vi "Write Resistor.vi"(8 "error in (no error)":errorcluster, 10 "Resistor Engine Refs in":T1 {"RT IDs"."Slot #" max=15; "RT IDs"."Chip Address (A2 A1 A0)" max=7; "RT Block Data Refs"."Data Reference" format="%.0x"}, 11 "DMA FIFO Ref in":refnum<k20>) -> (0 "error out":errorcluster, 2 "Resistor Engine Refs out":T1 {"RT IDs"."Slot #" max=15; "RT IDs"."Chip Address (A2 A1 A0)" max=7; "RT Block Data Refs"."Data Reference" format="%.0x"}, 3 "DMA FIFO Ref out":refnum<k20>)   [LabVIEW 2014, in "SLSC configuration Engine.lvlib"]
uses:
  SLSC configuration Engine.lvlib
  Type Defs/RT Engine Refs.ctl
  Shared/Type Defs/RT IDs.ctl
  Shared/SPI Utility/Slot #.ctl
  Shared/MCP23S17/Chip Address.ctl
  <vilib>/NI Veristand/Custom Device API/Block Data Reference.ctl
  <vilib>/NI Veristand/Custom Device API/Data Reference.ctl
  <vilib>/NI Veristand/Custom Device API/Global Data Refs.vi
  <vilib>/Utility/error.llb/Error Cluster From Error Code.vi
  <vilib>/rvi/errors/niLvFpgaAdjustHostInterfaceError.vi
  <vilib>/rvi/interface/nirviMethod/nirviMethod.xnode
  <vilib>/NI Veristand/Custom Device API/Custom Device API.lvlib
  <vilib>/FPGAPlugInAG/Dynamic/niLvFpga_WriteFifo_Dynamic.vi
  <vilib>/rvi/errors/niLvFpgaMergeErrorWithErrorCode.vi
  Shared/SLSC configuration Shared.lvlib
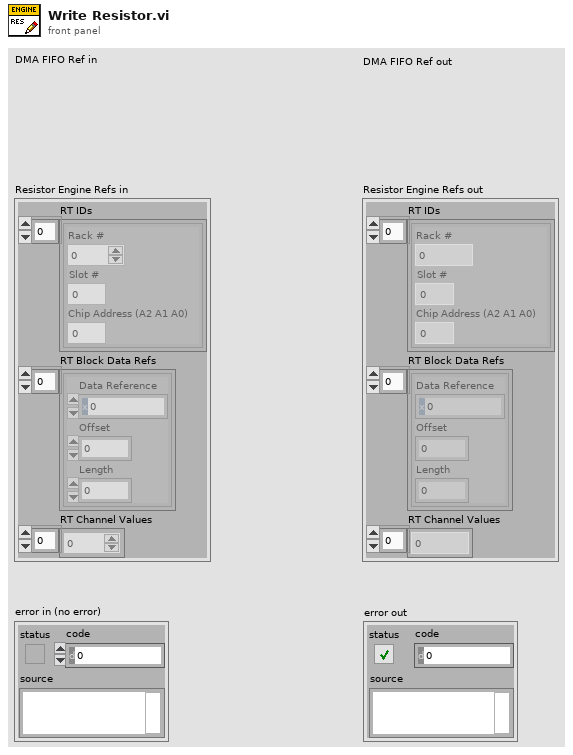
[diagram p1: front panel]
types:
  T1 = typedef "SLSC configuration Engine.lvlib/RT Engine Refs.ctl" = cluster{"RT IDs":T2[], "RT Block Data Refs":T5[], "RT Channel Values":dbl[]}
  T2 = typedef "SLSC configuration Shared.lvlib/RT IDs.ctl" = cluster{"Rack #":u8, "Slot #":T3, "Chip Address (A2 A1 A0)":T4}
  T3 = typedef "SLSC configuration Shared.lvlib/Slot #.ctl" = u8
  T4 = typedef "SLSC configuration Shared.lvlib/Chip Address.ctl" = u8
  T5 = typedef "Custom Device API.lvlib/Block Data Reference.ctl" = cluster{"Data Reference":T6, "Offset":i32, "Length":i32}
  T6 = typedef "Custom Device API.lvlib/Data Reference.ctl" = i32
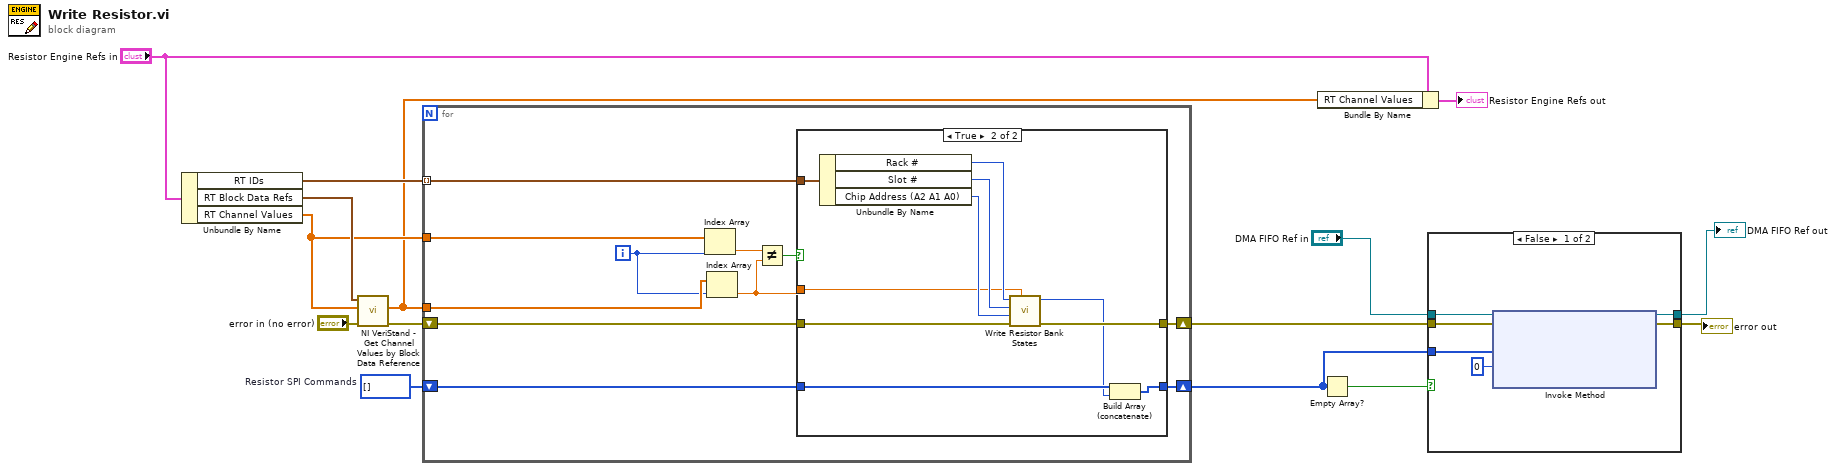
[diagram p0: block diagram]
diagram:
  w7 = u64[] []  # Resistor SPI Commands
  n1 = Unbundle By Name("Resistor Engine Refs in") -> ("RT IDs"=w12:T2[], "RT Block Data Refs"=w15:T5[], "RT Channel Values"=w10:dbl[])
  n2 = call <vilib>:"NI VeriStand - Get Channel Values by Block Data Reference.vi"("error in (no error)"="error in (no error)", "Values Array in"=w10, "Block Data Ref"=w15) -> ("error out"=w13:errorcluster, "Values Array out"=w9:dbl[])  [unwired: 6 in, 1 out]
  n3 = for {
    shift-right: [w20] -> w6
    shift-left: w13 -> [w22]
    tunnel: w12 -> [w23] mode=indexing
    tunnel: w9 -> [w25]
    tunnel: w10 -> [w26]
    shift-right: [w17] -> w3
    shift-left: w7 -> [w18]
    i -> [w16]
    n4 = Index Array(array=w26, index=w16) -> (element=w24:dbl)
    n5 = Index Array(array=w25, index=w16) -> (element=w21:dbl)
    n6 = Not Equal?(x=w24, y=w21) -> (x != y?=w19:bool)
    n7 = case shown="True" w19 {
      tunnel: w23 -> [_ w38]
      tunnel: w22 -> [w28 w37]
      tunnel: w21 -> [_ w29]
      tunnel: [w28 w33] -> w20
      tunnel: w18 -> [w27 w32]
      tunnel: [w27 w30] -> w17
      frame False {
      }
      frame True {
        n8 = Unbundle By Name(w38) -> ("Rack #"=w36:u8, "Slot #"=w35:T3, "Chip Address (A2 A1 A0)"=w34:T4)
        n9 = call "Write Resistor Bank States.vi"("Resistance (Ohms)"=w29, "error in (no error)"=w37, "Chip Address (A2 A1 A0)"=w34, "Slot #"=w35, "Rack #"=w36) -> ("error out"=w33:errorcluster, "FIFO SPI Message"=w31:u64)  [unwired: 4 in, 1 out]
        n10 = Build Array (concatenate)(w32, w31) -> (w30:u64[])
      }
    }
  }
  n11 = Bundle By Name(cluster="Resistor Engine Refs in", "RT Channel Values"=w9) -> (→"Resistor Engine Refs out":T1)
  n12 = Empty Array?(array=w3) -> (empty?=w5:bool)
  n13 = case shown="False" w5 {
    tunnel: "DMA FIFO Ref in" -> [w44 w45]
    tunnel: w6 -> [w42 w46]
    tunnel: [w41 w46] -> w4
    tunnel: w3 -> [w40 _]
    tunnel: [w39 w45] -> w1
    frame False {
      n14 = xnode "Invoke Method"("FPGA VI Reference In"=w44, "error in"=w42, "Data"=w40, "Timeout (ms)"=0) -> ("FPGA VI Reference Out"=w39:refnum<k20>, "error out"=w41:errorcluster)  [unwired: 1 out]
    }
    frame True {
    }
  }
  "error out" <- w4
  "DMA FIFO Ref out" <- w1
